vi "API_Get Last Error.vi"(8 "错误输入（无错误）":errorcluster) -> (0 "错误输出":errorcluster)   [LabVIEW 2011, in "API.lvlib"]
uses:
  API.lvlib
  kernel32.dll
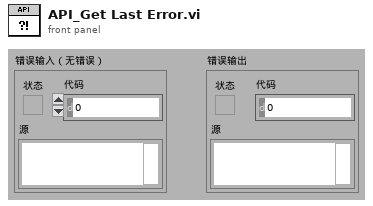
[diagram p1: front panel]
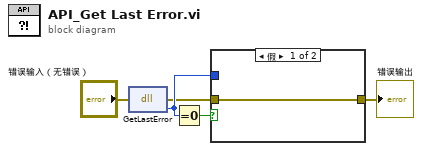
[diagram p0: block diagram]
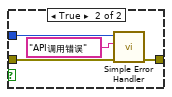
[diagram p2: hidden frame]
diagram:
  n1 = dll-call lib="kernel32.dll" fn="GetLastError"(error in="错误输入（无错误）") -> (error out=w2:errorcluster, "return type"=w3:u32)  [unwired: 2 in, 1 out]
  n2 = Equal To 0?(x=w3) -> (x = 0?=w4:bool)
  n3 = case shown="假" w4 {
    tunnel: w3 -> [_ w10]
    tunnel: w2 -> [w6 w8]
    tunnel: [w6 w7] -> w1
    frame False {
    }
    frame True {
      n4 = call <vilib>:"Simple Error Handler.vi"("error code (no error:0)"=w10, "error source (\" \")"="API调用错误" ("error source (\" \")"), "error in (no error)"=w8) -> ("error out"=w7:errorcluster)  [unwired: 2 in, 4 out]
    }
  }
  "错误输出" <- w1
